vi "Actor Core.vi"(8 "error in":errorcluster, 11 "Camera Controller in":refnum<class "Camera Controller.lvclass">) -> (0 "error out":errorcluster, 3 "Actor out":refnum<class "Actor.lvclass">)   [LabVIEW 2019, in "Camera Controller.lvlib" / "Camera Controller.lvclass"]
doc: "(<B>Filename</B>: Actor Framework.lvlib:Actor.lvclass:Actor Core.vi)\n\nReceives messages to the actor, reacts to them, and initiates any error handling that may shut the actor down.\n\nDescendant classes may override this VI to append parallel tasks for the actor to complete while it handles messages. Overrides use the Call Parent Method node."
uses:
  Camera Controller.lvclass
  <vilib>/vision/Image Controls.llb/IMAQ Image.ctl
  <vilib>/ActorFramework/Message Enqueuer/Message Enqueuer.lvclass
  TypeDef/Output Data.ctl
  TypeDef/CameraControllerParameters.ctl
  TypeDef/Initialize Data CC.ctl
  <vilib>/ActorFramework/Actor/Actor.lvclass
  Image Acquisition/Image Acquisition/Image Acquisition.lvclass
  Image Acquisition/Image Acquisition Messages/Image Acqusition Setup IA Msg/Image Acqusition Setup IA Msg.lvclass
  Image Acquisition/Image Acquisition Messages/Part Name IA Msg/Part Name IA Msg.lvclass
  Image Acquisition/Image Acquisition Messages/Run IA Msg/Run IA Msg.lvclass
  Image Acquisition/Image Acquisition Messages/State Message IA Msg/State Message IA Msg.lvclass
  <vilib>/ActorFramework/Message Enqueuer/Message Priority.ctl
  <vilib>/ActorFramework/Stop Msg/Stop Msg.lvclass
  SubVI/Image Trigger Global Count.vi
  Image Acquisition/Image Acquisition Messages/Camera Setup IA Msg/Camera Setup IA Msg.lvclass
  C:/Program Files/National Instruments/LabVIEW 2019/vi.lib/ActorFramework/Actor/Actor.lvclass
panel:
  out "Camera Controller ID":i32
  out "Error Message":string
  out "Image Array Counter":u64
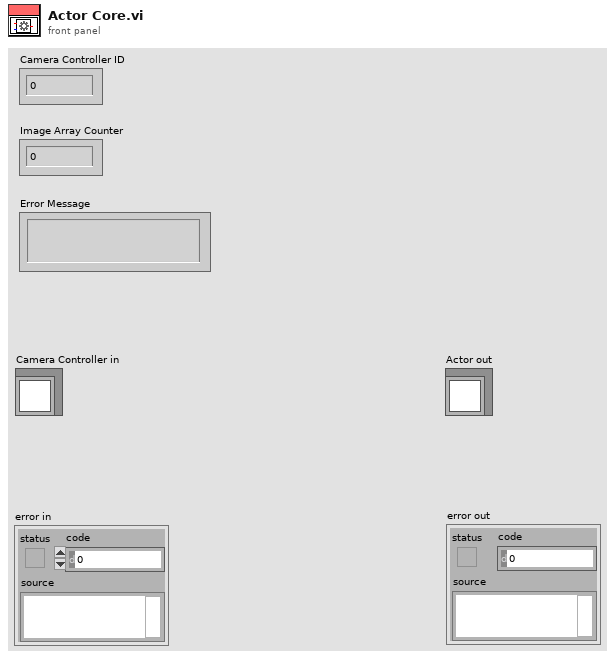
[diagram p1: front panel]
types:
  T1 = enum32{"invalid app kind", "Development System", "Run Time System", "Student Edition", "Embedded LabVIEW", "Evaluation", "Custom"}
  T2 = cluster{"Camera Id":i32, "Camera Name":string, "Exposure Time":i32, "AOI":i32[]}
  T3 = enum32{"Invalid", "Standard", "Closed", "Hidden", "Minimized", "Maximized"}
  T4 = typedef "Actor Framework.lvlib/Message Enqueuer.lvclass/Message Priority.ctl" = enum16{"Low", "Normal", "High"}
  T5 = cluster{"State":string, "Image File path":cluster{"Path":path, "Camera ID":i32}[]}
  T6 = cluster{"Image Acquisition ID":i32, "IA JSON File Path":path}
  T7 = typedef "Camera Controller.lvlib/Camera Controller.lvclass/Initialize Data CC.ctl" = cluster{"Core":cluster{"Current VI Reference":refnum<vi>, "Close Panel on Exit?":bool}, "CC ID":i32, "Part name":string, "Number of active cameras":i32[], "IA Camera names":string[], "Image count array":i32[][], "Diagnostics Child ID":i32, "Number of cameras":i32, "Image array":T8[][], "LiveMode":bool, "RecieversID":i32[], "Active Camera ID":i32[], "Enqueuer":cluster{"Caller Enqueuer":refnum<class "Message Enqueuer.lvclass">, "Nested Actor's Enqueuer":refnum<class "Message Enqueuer.lvclass">[], "Reciever Enqueuer ":cluster{"Reciever Enqueuers":refnum<class "Message Enqueuer.lvclass">, "Recievers Name":string, "Recievers ID":i32}[]}, "Image Array Counter":u64, "Images Recieved count":u64[], "All Camera Diagnostics":bool, "Output Data":T9, "Camera Setup":cluster{"Camera ID":i32, "Exposure time":i32}[], "Setup Response Received Count":u64, "Send Error to Caller":bool, "Camera Info Recieved":i32, "CameraControllerParameters":T10, "CurrentPartDetails":cluster{"PartName":string, "CameraIDs":i32[], "ReceiverSequence":cluster{"ReceiverName":string, "ReceiverID":i32, "NoOfActiveCameras":i32}[]}, "Run Info":cluster{"State":string, "Image File path":cluster{"Path":path, "Camera ID":i32}[]}, "Active Light Camera Name":string, "Captured Image Info":cluster{"Image out":T8, "Camera Location":string, "Count":u64, "RecieverSequence":cluster{"RecieverID":dbl, "Index":dbl}[]}, "Current Steps":string, "CurrentReceiverSequence":cluster{"ReceiverName":string, "ReceiverID":i32, "NoOfActiveCameras":i32}[], "Status Ack":cluster{"State":string, "Status":string}[]}
  T8 = typedef "IMAQ Image.ctl" = refnum<image>
  T9 = typedef "Camera Controller.lvlib/Camera Controller.lvclass/Output Data.ctl" = cluster{"Launch Handshake":cluster{"Actor Enqueuer Refnum":refnum<class "Message Enqueuer.lvclass">, "Actor core Refnum":refnum<vi>, "Actor Name":string}, "Launch Clear":bool, "Part Name":string, "Image Trigger Count":u64, "Image Array":T8[], "CamOpticsDiagnosticsResult":cluster{"Light Camera  Name":string, "Diagnosed Image":T8, "Dust Percentage":dbl, "Result":bool}, "State Ack":cluster{"State Message":string, "Status":string}, "Error Handler":string, "Camera Information":cluster{"Camera Id":i32, "Camera Name":string, "Exposure Time":i32, "AOI":i32[]}[], "Number of Active Camera":i32}
  T10 = typedef "Camera Controller.lvlib/Camera Controller.lvclass/CameraControllerParameters.ctl" = cluster{"CameraControllerParameters":cluster{"ID":i32, "FrontPanelOpen":bool, "NoOfCameras":i32, "CameraID":i32[], "NoOfReceivers":i32, "Diagnostics":cluster{"Path":string, "LightCameraSequence":cluster{"Name":string, "CameraID":i32, "LightID":i32}[], "Delaytime":dbl, "DecisitionParameters":cluster{"Range":i32[], "AcceptancePercentage":i32[], "Comparison":string[], "AcceptableBlackBinValue":i32}, "DiagnosticReceiverSequence":cluster{"ReceiverName":string, "ReceiverID":i32}}, "PartsList":cluster{"PartName":string, "CameraIDs":i32[], "ReceiverSequence":cluster{"ReceiverName":string, "ReceiverID":i32, "NoOfActiveCameras":i32}[]}[]}, "PartName":string[]}
  T11 = cluster{"Reciever Enqueuers":refnum<class "Message Enqueuer.lvclass">, "Recievers Name":string, "Recievers ID":i32}[]
  T12 = cluster{"Reciever Enqueuers":refnum<class "Message Enqueuer.lvclass">, "Reciever Name":string, "Reciever ID":i32}
  T13 = cluster{"Camera Id":i32, "Camera Name":string, "Exposure Time":i32, "AOI":i32[]}[]
  T14 = cluster{"ReceiverName":string, "ReceiverID":i32, "NoOfActiveCameras":i32}[]
  T15 = cluster{"ReceiverName":string, "ReceiverID":i32, "NoOfCameras":i32}
  T16 = cluster{"PartName":string, "CameraIDs":i32[], "ReceiverSequence":cluster{"ReceiverName":string, "ReceiverID":i32, "NoOfActiveCameras":i32}[]}[]
  T17 = cluster{"PartName":string, "CameraIDs":i32[], "ReceiverSequence":cluster{"ReceiverName":string, "ReceiverID":i32, "NoOfActiveCameras":i32}[]}
  T18 = cluster{"ReceiverName":string, "ReceiverID":i32, "NoOfCameras":i32}[]
  T19 = cluster{"Name":string, "CameraID":i32, "LightID":i32}[]
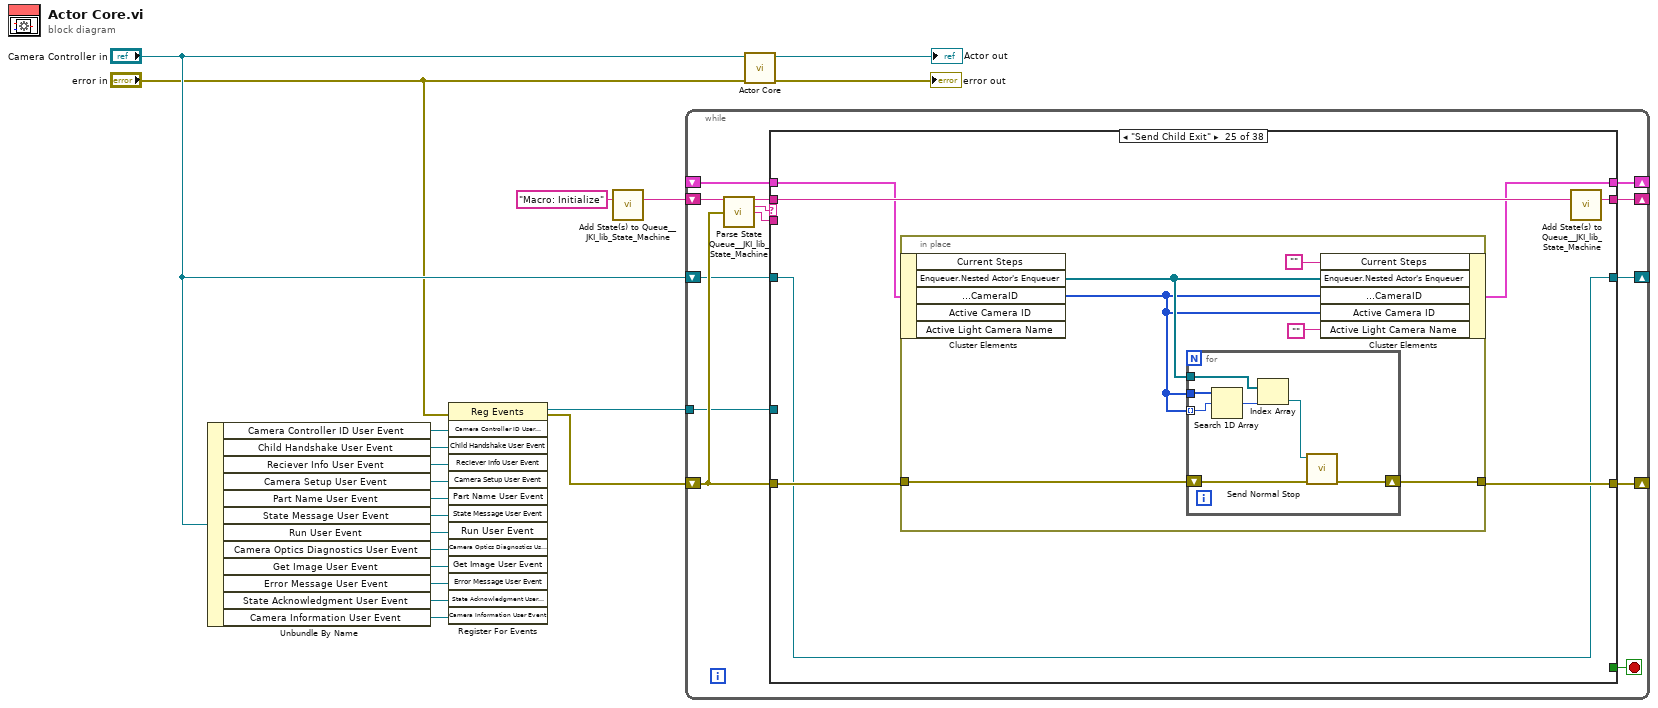
[diagram p0: block diagram]
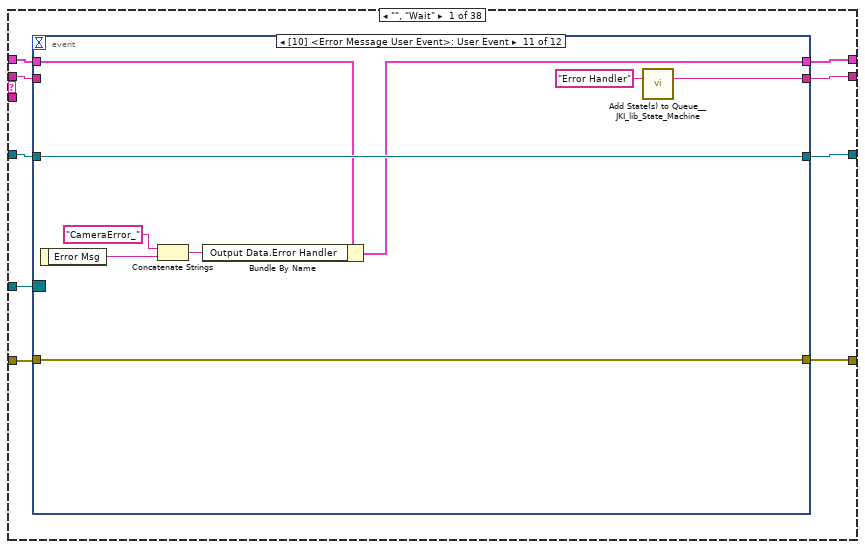
[diagram p2: hidden frame]
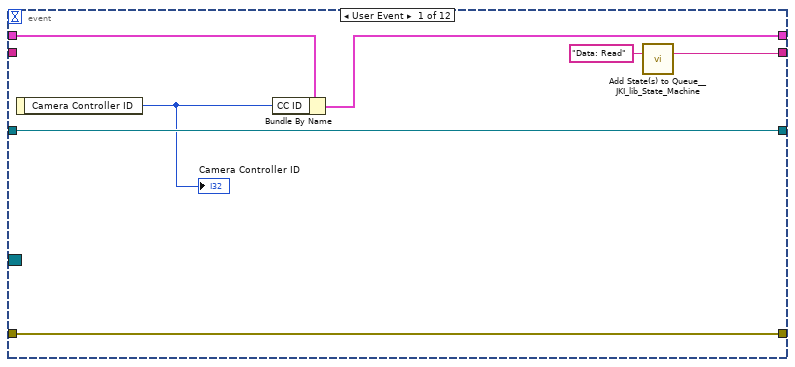
[diagram p3: hidden frame]
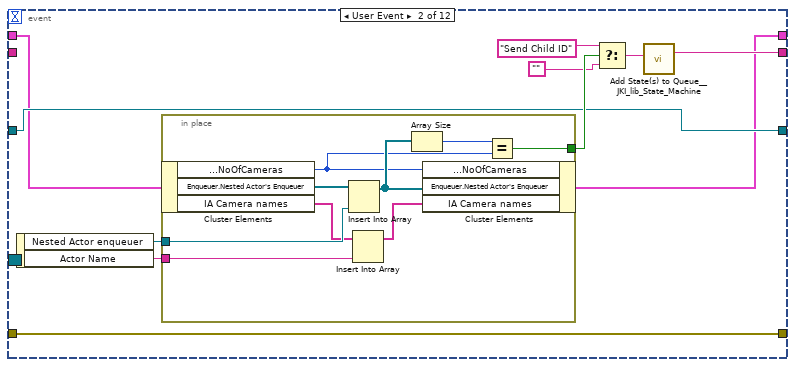
[diagram p4: hidden frame]
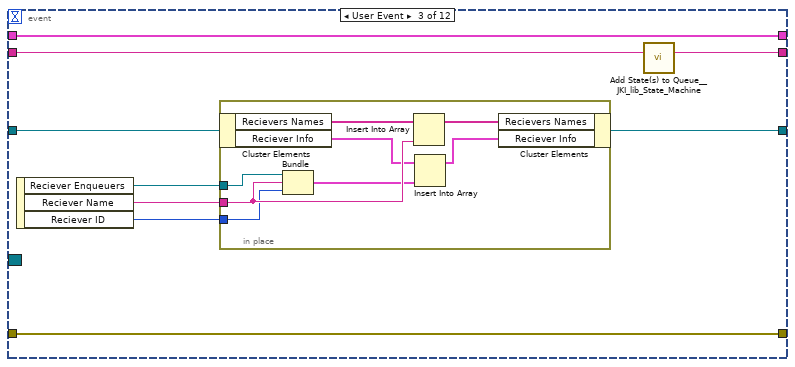
[diagram p5: hidden frame]
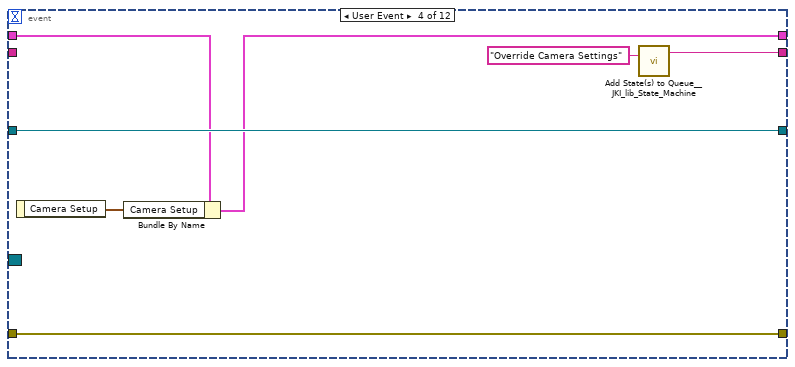
[diagram p6: hidden frame]
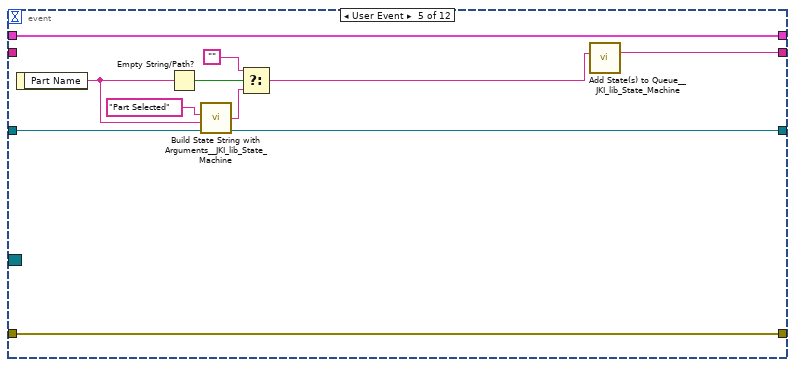
[diagram p7: hidden frame]
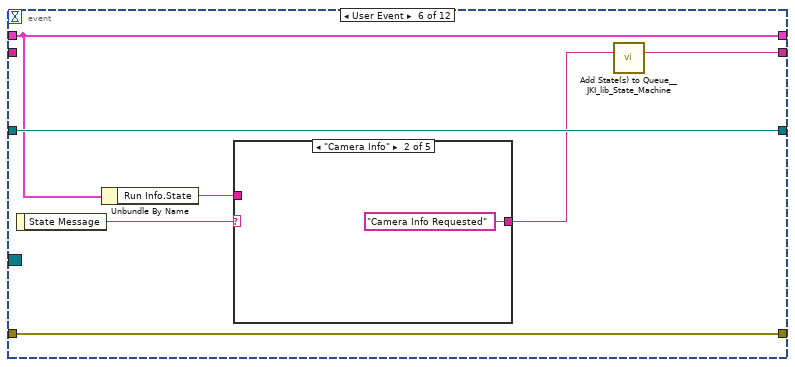
[diagram p8: hidden frame]
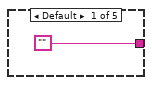
[diagram p9: hidden frame]
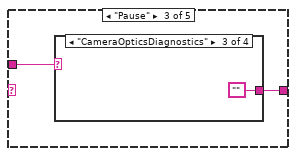
[diagram p10: hidden frame]
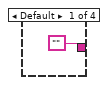
[diagram p11: hidden frame]
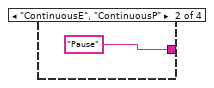
[diagram p12: hidden frame]
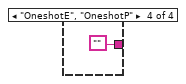
[diagram p13: hidden frame]
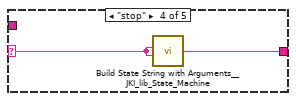
[diagram p14: hidden frame]
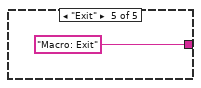
[diagram p15: hidden frame]
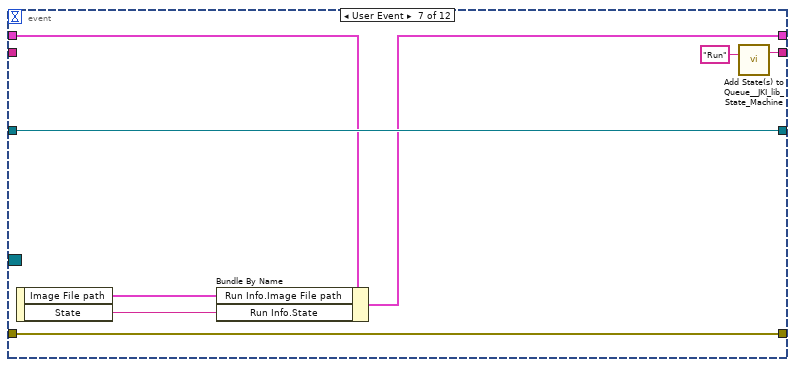
[diagram p16: hidden frame]
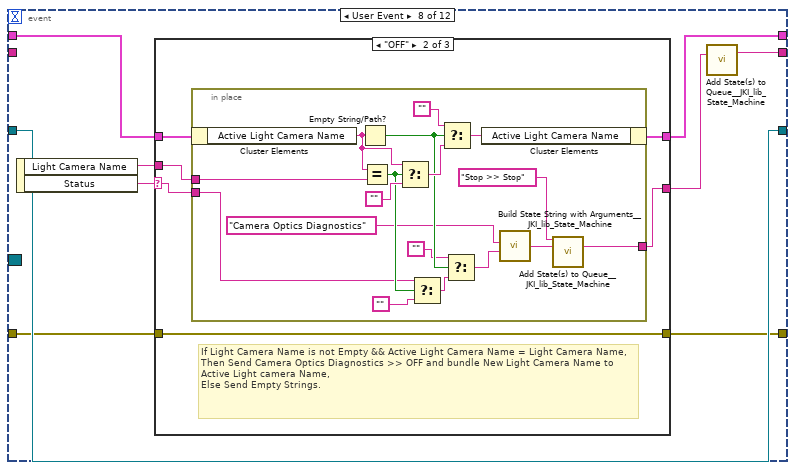
[diagram p17: hidden frame]
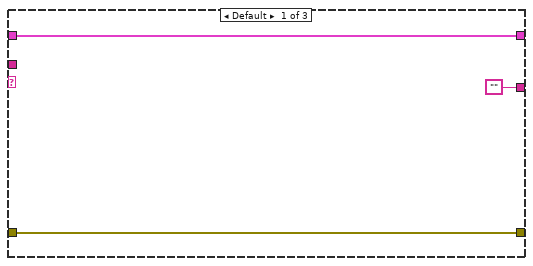
[diagram p18: hidden frame]
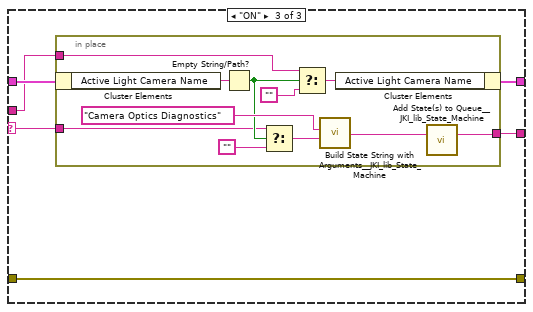
[diagram p19: hidden frame]
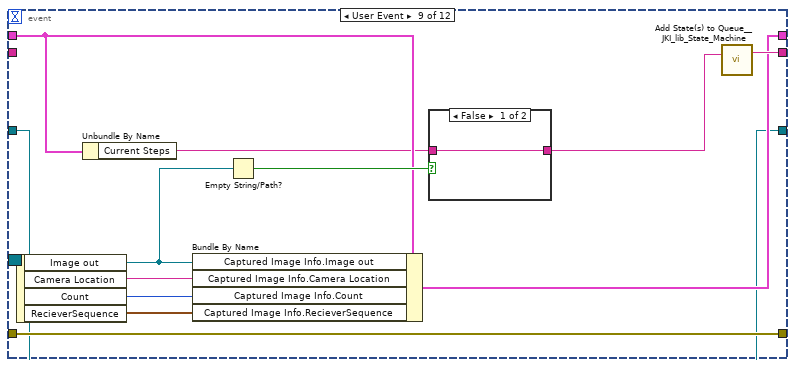
[diagram p20: hidden frame]
diagram:
  n1 = Unbundle By Name("Camera Controller in") -> ("Camera Controller ID User Event"=w16:refnum<user-event>, "Child Handshake User Event"=w15:refnum<user-event>, "Reciever Info User Event"=w14:refnum<user-event>, "Camera Setup User Event"=w13:refnum<user-event>, "Part Name User Event"=w12:refnum<user-event>, "State Message User Event"=w11:refnum<user-event>, "Run User Event"=w10:refnum<user-event>, "Camera Optics Diagnostics User Event"=w9:refnum<user-event>, "Get Image User Event"=w8:refnum<user-event>, "Error Message User Event"=w7:refnum<user-event>, "State Acknowledgment User Event"=w6:refnum<user-event>, "Camera Information User Event"=w1:refnum<user-event>)
  n2 = register-events(error in="error in", w16, w15, w14, w13, w12, w11, w10, w9, w8, w7, w6, w1) -> (reference out=w4:refnum<event-registration>, error out=w5:errorcluster)  [unwired: 1 in]
  n3 = call <vilib>:"Add State(s) to Queue__JKI_lib_State_Machine.vi"("State(s) in (\"\")"="Macro: Initialize") -> ("States Out"=w19:string)  [unwired: 14 in]
  n4 = while {
    shift-right: [w26] -> _
    shift-left: _ -> [w25]
    shift-right: [w29] -> _
    shift-left: w5 -> [w24]
    shift-right: [w28] -> _
    shift-left: w19 -> [w30]
    tunnel: w4 -> [w23]
    shift-right: [w21] -> _
    shift-left: "Camera Controller in" -> [w22]
    stop <- w27 stop-if-true
    n5 = call <vilib>:"Parse State Queue__JKI_lib_State_Machine.vi"("State Queue"=w30, "Error In (no error)"=w24) -> ("Remaining States"=w32:string, "Current State"=w33:string, "Arguments"=w31:string)  [unwired: 11 in]
    n6 = case shown="\"Send Child Exit\"" w33 {
      selector: w33 -> [_ _ w255 _ _ _ _ _ _ _ _ _ _ _ _ _ _ _ _ _ _ _ _ _ _ _ _ _ _ _ _ _ _ _ _ _ _ _]
      tunnel: w32 -> [w42 w253 w259 w278 w289 w307 w312 w317 _ w356 w361 w366 w373 w385 w412 w418 w431 w436 w443 w483 w509 _ w571 w595 w629 w647 w659 w675 _ w712 w717 _ w762 w767 _ w790 w806 w828]
      tunnel: w31 -> [_ _ _ _ _ _ _ _ _ _ _ _ w368 w379 _ _ _ _ _ w459 _ _ _ w591 _ _ _ _ _ _ _ w719 _ _ _ _ _ _]
      tunnel: w25 -> [w40 w250 w257 w269 w282 w305 w309 _ w325 w352 w358 w364 w371 w381 w409 w415 w429 w433 w439 w464 w504 w535 w566 w592 w625 w644 w648 w662 w691 w705 w714 w722 w753 w764 w773 w787 w799 w821]
      tunnel: [w39 w251 w261 w275 errorcluster {"status"=FALSE, "code"=0, "source"=""} ("error out") w304 w310 w314 w330 w351 w359 w363 w369 w382 w410 w416 w420 w434 w440 w465 w506 w536 w568 w593 w626 w645 w656 w672 w692 w709 w715 w720 w750 w765 w776 w788 w803 w825] -> w29
      tunnel: w24 -> [w38 w251 w260 w275 w281 w304 w310 w314 w331 w353 w359 w363 w370 w383 w410 w416 w421 w434 w441 w466 w507 w537 w569 w589 w627 w645 w657 w673 w693 w710 w715 w720 w754 w765 w777 w788 w804 w826]
      tunnel: [w41 w252 w258 w277 w288 w306 w311 w316 w332 w355 w360 w365 w372 w384 w411 w417 w430 w435 w442 w482 w508 w538 w570 w594 w628 w646 w658 w674 w694 w711 w716 w724 w761 w766 w778 w789 w805 w827] -> w28
      tunnel: [_ _ _ _ _ TRUE _ _ _ _ _ _ _ _ _ _ _ _ _ _ _ _ _ _ _ _ _ _ _ _ _ _ _ _ _ _ _ _] -> w27
      tunnel: [w37 w250 w257 w276 w282 w305 w309 w315 w324 w352 w358 w364 w371 w381 w409 w415 w429 w433 w438 w477 w503 w534 w565 w586 w624 w644 w648 w661 w691 w705 w714 w721 w753 w764 w772 w787 w798 w820] -> w26
      tunnel: w23 -> [w36 _ _ _ _ _ _ _ _ w346 _ _ _ _ _ _ w419 _ _ _ _ _ _ w587 _ _ _ _ _ _ _ _ _ _ _ _ _ _]
      tunnel: w22 -> [w35 w249 w254 w266 w285 w302 w308 w313 w329 w350 w357 w362 w367 w378 w408 w413 w422 w432 w437 w478 w505 w533 w567 w590 w623 w643 w650 w660 w688 w708 w713 w723 w749 w763 w774 w786 w802 w824]
      tunnel: [w34 w249 w254 w266 w284 w302 w308 w313 w329 w349 w357 w362 w367 w378 w408 w413 w422 w432 w437 w478 w505 w533 w567 w590 w623 w643 w649 w660 w688 w707 w713 w723 w748 w763 w775 w786 w801 w823] -> w21
      frame "", "Wait" {
        n7 = event shown="[10] <Error Message User Event>: User Event" {
          selector: w36 -> [_ _ _ _ _ _ _ _ _ _ _ _]
          dyn-events: _ -> [_ _ _ _ _ _ _ _ _ _ _ _]
          timeout: _ -> [_ _ _ _ _ _ _ _ _ _ _ _]
          tunnel: w42 -> [_ _ w75 _ _ _ _ _ _ _ _ w235]
          tunnel: [w49 w59 w76 w92 w101 w109 w129 w138 w192 w197 w226 w236] -> w41
          tunnel: w40 -> [w44 w51 w77 w89 w102 w105 w126 w134 w184 w199 w223 w234]
          tunnel: [w48 w60 w78 w93 w103 w110 w127 w130 w193 w206 w227 w237] -> w39
          tunnel: w38 -> [w48 w60 w78 w93 w103 w110 w127 w131 w193 w206 w227 w237]
          tunnel: [w43 w50 w77 w88 w102 w105 w123 w133 w188 w198 w222 w233] -> w37
          tunnel: w35 -> [w46 w52 w74 w91 w100 w108 w128 w132 w186 w205 w225 w228]
          tunnel: [w46 w52 w70 w91 w100 w108 w128 w132 w186 w205 w225 w228] -> w34
          event User Event {
            n8 = event-data() -> ("Camera Controller ID"=w45:i32)  [unwired: 1 in]
            "Camera Controller ID" <- w45
            n9 = Bundle By Name(cluster=w44, "CC ID"=w45) -> (w43:T7)
            n10 = call <vilib>:"Add State(s) to Queue__JKI_lib_State_Machine.vi"("State(s) in (\"\")"="Data: Read" ("State(s) in (\"\")")) -> ("States Out"=w49:string)  [unwired: 14 in]
          }
          event User Event {
            n11 = event-data() -> ("Nested Actor enqueuer"=w58:refnum<class "Message Enqueuer.lvclass">, "Actor Name"=w57:string)  [unwired: 1 in]
            n12 = in-place {
              in-place-border: w58 -> [w68]
              in-place-border: w57 -> [w66]
              in-place-border: [w61] -> w56
              n13 = in-place-cluster #1(w51) -> ("CameraControllerParameters.CameraControllerParameters.NoOfCameras"=w62:i32, "Enqueuer.Nested Actor's Enqueuer"=w69:refnum<class "Message Enqueuer.lvclass">[], "IA Camera names"=w67:string[])
              n14 = Insert Into Array(array=w69, new element=w68) -> (w63:refnum<class "Message Enqueuer.lvclass">[])  [unwired: 1 in]
              n15 = Insert Into Array(array=w67, new element=w66) -> (w65:string[])  [unwired: 1 in]
              n16 = Array Size(array=w63) -> (size(s)=w64:i32)
              n17 = in-place-cluster #1("CameraControllerParameters.CameraControllerParameters.NoOfCameras"=w62, "Enqueuer.Nested Actor's Enqueuer"=w63, "IA Camera names"=w65) -> (w50:T7)
              n18 = Equal?(x=w64, y=w62) -> (x = y?=w61:bool)
            }
            n19 = Select(t="Send Child ID", s=w56, f="") -> (s? t:f=w55:string)
            n20 = call <vilib>:"Add State(s) to Queue__JKI_lib_State_Machine.vi"("State(s) in (\"\")"=w55) -> ("States Out"=w59:string)  [unwired: 14 in]
          }
          event User Event {
            n21 = event-data() -> ("Reciever Enqueuers"=w73:refnum<class "Message Enqueuer.lvclass">, "Reciever Name"=w72:string, "Reciever ID"=w71:i32)  [unwired: 1 in]
            n22 = in-place {
              in-place-border: w73 -> [w84]
              in-place-border: w72 -> [w83]
              in-place-border: w71 -> [w82]
              n23 = in-place-cluster #2(w74) -> ("Recievers Names"=w86:string[], "Reciever Info"=w80:T11)
              n24 = Bundle("Reciever Enqueuers"=w84, "Reciever Name"=w83, "Reciever ID"=w82) -> (w81:T12)  [unwired: 1 in]
              n25 = Insert Into Array(array=w86, new element=w83) -> (w85:string[])  [unwired: 1 in]
              n26 = Insert Into Array(array=w80, new element=w81) -> (w79:T11)  [unwired: 1 in]
              n27 = in-place-cluster #2("Recievers Names"=w85, "Reciever Info"=w79) -> (w70:refnum<class "Camera Controller.lvclass">)
            }
            n28 = call <vilib>:"Add State(s) to Queue__JKI_lib_State_Machine.vi"("State(s) in (\"\")"=w75) -> ("States Out"=w76:string)  [unwired: 14 in]
          }
          event User Event {
            n29 = event-data() -> ("Camera Setup"=w90:cluster{"Camera ID":i32, "Exposure time":i32}[])  [unwired: 1 in]
            n30 = Bundle By Name(cluster=w89, "Camera Setup"=w90) -> (w88:T7)
            n31 = call <vilib>:"Add State(s) to Queue__JKI_lib_State_Machine.vi"("State(s) in (\"\")"="Override Camera Settings" ("State(s) in (\"\")")) -> ("States Out"=w92:string)  [unwired: 14 in]
          }
          event User Event {
            n32 = event-data() -> ("Part Name"=w96:string)  [unwired: 1 in]
            n33 = Empty String/Path?(string/path=w96) -> (empty?=w98:bool)
            n34 = call <vilib>:"Build State String with Arguments__JKI_lib_State_Machine.vi"("Arguments (\"\")"=w96, "State"="Part Selected" ("State(s) in (\"\")")) -> ("State with Arguments"=w97:string)  [unwired: 4 in]
            n35 = Select(t="", s=w98, f=w97) -> (s? t:f=w94:string)
            n36 = call <vilib>:"Add State(s) to Queue__JKI_lib_State_Machine.vi"("State(s) in (\"\")"=w94) -> ("States Out"=w101:string)  [unwired: 14 in]
          }
          event User Event {
            n37 = event-data() -> ("State Message"=w107:string)  [unwired: 1 in]
            n38 = Unbundle By Name(w105) -> ("Run Info.State"=w104:string)
            n39 = case shown="\"Camera Info\"" w107 {
              selector: w107 -> [_ _ _ w119 _]
              tunnel: ["" "Camera Info Requested" ("State with Arguments") w113 w120 "Macro: Exit"] -> w106
              tunnel: w104 -> [_ _ w114 _ _]
              frame Default {
              }
              frame "Camera Info" {
              }
              frame "Pause" {
                n40 = case shown="\"CameraOpticsDiagnostics\"" w114 {
                  tunnel: ["" "Pause" "" ""] -> w113
                  frame Default {
                  }
                  frame "ContinuousE", "ContinuousP" {
                  }
                  frame "CameraOpticsDiagnostics" {
                  }
                  frame "OneshotE", "OneshotP" {
                  }
                }
              }
              frame "stop" {
                n41 = call <vilib>:"Build State String with Arguments__JKI_lib_State_Machine.vi"("Arguments (\"\")"=w119, "State"=w119) -> ("State with Arguments"=w120:string)  [unwired: 4 in]
              }
              frame "Exit" {
              }
            }
            n42 = call <vilib>:"Add State(s) to Queue__JKI_lib_State_Machine.vi"("State(s) in (\"\")"=w106) -> ("States Out"=w109:string)  [unwired: 14 in]
          }
          event User Event {
            n43 = event-data() -> ("Image File path"=w124:cluster{"Path":path, "Camera ID":i32}[], "State"=w125:string)  [unwired: 1 in]
            n44 = Bundle By Name(cluster=w126, "Run Info.Image File path"=w124, "Run Info.State"=w125) -> (w123:T7)
            n45 = call <vilib>:"Add State(s) to Queue__JKI_lib_State_Machine.vi"("State(s) in (\"\")"="Run" ("State(s) in (\"\")")) -> ("States Out"=w129:string)  [unwired: 14 in]
          }
          event User Event {
            n46 = event-data() -> ("Light Camera Name"=w136:string, "Status"=w135:string)  [unwired: 1 in]
            n47 = case shown="\"OFF\"" w135 {
              selector: w135 -> [_ w143 w167]
              tunnel: ["" w144 w166] -> w137
              tunnel: w134 -> [w141 w147 w170]
              tunnel: w136 -> [_ w146 w169]
              tunnel: [w141 w145 w168] -> w133
              tunnel: w131 -> [w139 w142 w165]
              tunnel: [w139 w142 w165] -> w130
              frame Default {
              }
              frame "OFF" {
                # "If Light Camera Name is not Empty && Active Light Camera Name = Light Camera Name,\nThen Send Camera Optics Diagnostics >> OFF and bundle New Light Camera Name to Active Light camera Name, \nElse Send Empty Strings."
                n48 = in-place {
                  in-place-border: w146 -> [w163]
                  in-place-border: [w148] -> w144
                  in-place-border: w143 -> [w153]
                  n49 = in-place-cluster #3(w147) -> ("Active Light Camera Name"=w160:string)
                  n50 = Empty String/Path?(string/path=w160) -> (empty?=w158:bool)
                  n51 = Equal?(x=w160, y=w163) -> (x = y?=w157:bool)
                  n52 = Select(t=w160, s=w157, f="") -> (s? t:f=w161:string)
                  n53 = Select(t=w153, s=w157, f="") -> (s? t:f=w156:string)
                  n54 = Select(t="" ("f"), s=w158, f=w161) -> (s? t:f=w162:string)
                  n55 = Select(t="" ("f"), s=w158, f=w156) -> (s? t:f=w152:string)
                  n56 = in-place-cluster #3("Active Light Camera Name"=w162) -> (w145:T7)
                  n57 = call <vilib>:"Build State String with Arguments__JKI_lib_State_Machine.vi"("Arguments (\"\")"=w152, "State"="Camera Optics Diagnostics" ("State(s) in (\"\")")) -> ("State with Arguments"=w150:string)  [unwired: 4 in]
                  n58 = call <vilib>:"Add State(s) to Queue__JKI_lib_State_Machine.vi"("State(s) in Front (\"\")"="Stop >> Stop" ("State(s) in (\"\")"), "State(s) in (\"\")"=w150) -> ("States Out"=w148:string)  [unwired: 13 in]
                }
              }
              frame "ON" {
                n59 = in-place {
                  in-place-border: w169 -> [w180]
                  in-place-border: w167 -> [w175]
                  in-place-border: [w171] -> w166
                  n60 = in-place-cluster #4(w170) -> ("Active Light Camera Name"=w181:string)
                  n61 = Empty String/Path?(string/path=w181) -> (empty?=w176:bool)
                  n62 = Select(t=w175, s=w176, f="") -> (s? t:f=w173:string)
                  n63 = Select(t=w180, s=w176, f="") -> (s? t:f=w178:string)
                  n64 = call <vilib>:"Build State String with Arguments__JKI_lib_State_Machine.vi"("Arguments (\"\")"=w173, "State"="Camera Optics Diagnostics" ("State(s) in (\"\")")) -> ("State with Arguments"=w172:string)  [unwired: 4 in]
                  n65 = in-place-cluster #4("Active Light Camera Name"=w178) -> (w168:T7)
                  n66 = call <vilib>:"Add State(s) to Queue__JKI_lib_State_Machine.vi"("State(s) in (\"\")"=w172) -> ("States Out"=w171:string)  [unwired: 14 in]
                }
              }
            }
            n67 = call <vilib>:"Add State(s) to Queue__JKI_lib_State_Machine.vi"("State(s) in (\"\")"=w137) -> ("States Out"=w138:string)  [unwired: 14 in]
          }
          event User Event {
            n68 = event-data() -> ("Image out"=w187:T8, "Camera Location"=w191:string, "Count"=w190:u64, "RecieverSequence"=w189:cluster{"RecieverID":dbl, "Index":dbl}[])  [unwired: 1 in]
            n69 = Unbundle By Name(w184) -> ("Current Steps"=w183:string)
            n70 = Bundle By Name(cluster=w184, "Captured Image Info.Image out"=w187, "Captured Image Info.Camera Location"=w191, "Captured Image Info.Count"=w190, "Captured Image Info.RecieverSequence"=w189) -> (w188:T7)
            n71 = Empty String/Path?(string/path=w187) -> (empty?=w185:bool)
            n72 = case shown="False" w185 {
              tunnel: w183 -> [w194 _]
              tunnel: [w194 ""] -> w182
              frame False {
              }
              frame True {
              }
            }
            n73 = call <vilib>:"Add State(s) to Queue__JKI_lib_State_Machine.vi"("State(s) in (\"\")"=w182) -> ("States Out"=w192:string)  [unwired: 14 in]
          }
          event User Event {
            n74 = event-data() -> ("Camera Id"=w201:i32, "Camera Name"=w204:string, "Exposure Time"=w202:i32, "AOI"=w203:i32[])  [unwired: 1 in]
            n75 = Bundle("Camera Id"=w201, "Camera Name"=w204, "Exposure Time"=w202, "AOI"=w203) -> (w200:T2)  [unwired: 1 in]
            n76 = in-place {
              in-place-border: w201 -> [w216]
              in-place-border: w200 -> [w217]
              in-place-border: [w208] -> w196
              n77 = in-place-cluster #5(w199) -> ("Active Camera ID"=w213:i32[], "Camera Info Recieved"=w212:i32, "Output Data.Camera Information"=w218:T13)
              n78 = Array Size(array=w213) -> (size(s)=w214:i32)
              n79 = Increment(x=w212) -> (x+1=w211:i32)
              n80 = Replace Array Subset(array=w218, new element=w217, index=w216) -> (w215:T13)
              n81 = Equal?(x=w214, y=w211) -> (x = y?=w210:bool)
              n82 = Select(t="Send Merged Camera Information", s=w210, f="") -> (s? t:f=w208:string)
              n83 = in-place-cluster #5("Active Camera ID"=w213, "Camera Info Recieved"=w211, "Output Data.Camera Information"=w215) -> (w198:T7)
            }
            n84 = call <vilib>:"Add State(s) to Queue__JKI_lib_State_Machine.vi"("State(s) in (\"\")"=w196) -> ("States Out"=w197:string)  [unwired: 14 in]
          }
          event User Event {
            n85 = event-data() -> ("Error Msg"=w220:string)  [unwired: 1 in]
            n86 = Concatenate Strings("CameraError_" ("string"), w220) -> (w219:string)
            n87 = Bundle By Name(cluster=w223, "Output Data.Error Handler"=w219) -> (w222:T7)
            n88 = call <vilib>:"Add State(s) to Queue__JKI_lib_State_Machine.vi"("State(s) in (\"\")"="Error Handler" ("State(s) in (\"\")")) -> ("States Out"=w226:string)  [unwired: 14 in]
          }
          event User Event {
            n89 = event-data() -> ("State"=w231:string, "Status"=w232:string)  [unwired: 1 in]
            n90 = Bundle("State"=w231, "Status"=w232) -> (w230:cluster{"State":string, "Status":string})  [unwired: 1 in]
            n91 = in-place {
              in-place-border: w230 -> [w238]
              in-place-border: [w240] -> w229
              n92 = in-place-cluster #6(w234) -> ("Active Camera ID"=w245:i32[], "Setup Response Received Count"=w244:u64, "Status Ack"=w248:cluster{"State":string, "Status":string}[])
              n93 = Array Size(array=w245) -> (size(s)=w246:i32)
              n94 = Increment(x=w244) -> (x+1=w243:u64)
              n95 = Replace Array Subset(array=w248, new element=w238) -> (w247:cluster{"State":string, "Status":string}[])  [unwired: 1 in]
              n96 = Equal?(x=w246, y=w243) -> (x = y?=w242:bool)
              n97 = Select(t="Send State Ack", s=w242, f="") -> (s? t:f=w240:string)
              n98 = in-place-cluster #6("Active Camera ID"=w245, "Setup Response Received Count"=w243, "Status Ack"=w247) -> (w233:T7)
            }
            n99 = call <vilib>:"Add State(s) to Queue__JKI_lib_State_Machine.vi"("State(s) in Front (\"\")"=w229, "State(s) in (\"\")"=w235) -> ("States Out"=w236:string)  [unwired: 13 in]
          }
        }
      }
      frame "---------- Core ----------" {
        n100 = call <vilib>:"Add State(s) to Queue__JKI_lib_State_Machine.vi"("State(s) in (\"\")"=w253) -> ("States Out"=w252:string)  [unwired: 14 in]
      }
      frame Default {
        w264 = 42 items=["No error", "Argument error", "Memory is full", "Out of zone", "End of file", "File already open", "Generic file I/O error", "File not found", "File permission error", "Disk is full", "Duplicate path", "Too many files open", "System feature not enabled", "Resource file not found", "Cannot add resource", "Resource not found", "Image not found", "Image memory error", "Pen does not exist", "Config type invalid", "Config token not found", "Config parse error", "Config memory error", "Bad external code format", "Bad external code offset", "External code not present", "Null window", "Destroy window error", "Null menu", "Print aborted", "Bad print record", "Print driver error", "Windows error during printing", "Memory error during printing", "Print dialog error", "Generic print error", "Invalid device refnum", "Device not found", "Device parameter error", "Device unit error", "Cannot open device", "Device call aborted", "Generic error", "Cancelled by user", "Object ID too low", "Object ID too high", "Object not in heap", "Unknown heap", "Unknown object (invalid DefProc)", "Unknown object (DefProc not in table)", "Message out of range", "Invalid (null) method", "Unknown message", "Manager call not supported", "Bad address", "Network operation in progress", "Network operation timed out", "Connection is busy", "Network attribute not supported", "Network error", "Address in use", "System out of memory", "Connection aborted", "Connection refused", "Not connected", "Already connected", "Connection closed", "Initialization error (interapplication manager)", "Bad occurrence", "Wait on unbound occurrence handler", "Occurrence queue overflow", "Datalog type conflict", "Unused", "Unrecognized type (interapplication manager)", "Memory corrupt", "Failed to make temporary DLL", "Old CIN version", "Drag socket not found", "Failed to load drop-object", "Failed to register OLE object", "Failed to release OLE object", "Format specifier type mismatch", "Unknown format specifier", "Too few format specifiers", "Too many format specifiers", "Scan failed", "Newer CIN version", "Error converting to variant", "Runtime menu error", "Password tampered", "Variant attribute not found", "Incompatible variant data type", "Event data is not available", "Event Store is not present", "Occurrence is not found", "Event Queue is not created", "Event info is not available", "Refnum passed is NULL", "Error retrieving Class GUID", "Error retrieving CoClass GUID", "Error retrieving TypeLib GUID.", "Bad built application magic bytes.", "Specific driver is different from the specific driver associated with the Logical Name.", "There is no session opened to the class driver.", "Max Error", "MAX - Error with config objects", "MAX - Error loading configuration", "MAX - Group not supported"]
        # "Current State"
        # "Do not delete, rename, or modify this frame.\n(this is used to capture unhandled states and typos)"
        # "Handle mistyped state name (developer tool)"
        n101 = Format Into String(format string="Software Exception: Unhandled State \"%s\"." ("message"), error in=w260, w255) -> (resulting string=w263:string, error out=w262:errorcluster)  [unwired: 1 in]
        n102 = call <vilib>:"Error Cluster From Error Code.vi"("show call chain? (False)"=TRUE, "error in (no error)"=w262, "error message (\"\")"=w263, "error code (0)"=w264) -> ("error out"=w261:errorcluster)  [unwired: 5 in]
        n103 = call <vilib>:"Add State(s) to Queue__JKI_lib_State_Machine.vi"("State(s) in (\"\")"=w259) -> ("States Out"=w258:string)  [unwired: 14 in]
      }
      frame "Initialize Core Data" {
        # "Do not delete, rename, or modify this frame.\n(this is used to determine panel behavior on exit)"
        # "originally closed?"
        # "exe?"
        # "If panel starts closed or is an EXE, then close it when we exit"
        n104 = property class="VI"() -> ("Front Panel.Open"=w274:bool)  [unwired: 2 in, 2 out]
        n105 = property class="App"() -> ("App.Kind"=w273:T1)  [unwired: 2 in, 2 out]
        n106 = control-ref of="Current VI Reference"() -> (w267:refnum<vi>)
        n107 = Not(x=w274) -> (.not. x?=w271:bool)
        n108 = Equal?(x=w273, y=T1."Run Time System" ("Application:Kind")) -> (x = y?=w270:bool)
        n109 = Or(x=w271, y=w270) -> (x .or. y?=w268:bool)
        n110 = Bundle By Name(cluster=w269, "Core.Current VI Reference"=w267, "Core.Close Panel on Exit?"=w268) -> (w276:T7)
        n111 = call <vilib>:"Add State(s) to Queue__JKI_lib_State_Machine.vi"("State(s) in (\"\")"=w278) -> ("States Out"=w277:string)  [unwired: 14 in]
      }
      frame "Error Handler" {
        # "Clear error"
        n112 = case shown="No Error" w281 {
          selector: w281 -> [_ w301]
          tunnel: w282 -> [w291 w299]
          tunnel: [w290 w297] -> w280
          frame No Error {
            n113 = Unbundle By Name(w291) -> ("Output Data"=w290:T9)
          }
          frame Error {
            n114 = Unbundle By Name(w301) -> ("code"=w300:i32)
            n115 = Unbundle By Name(w299) -> ("Output Data"=w298:T9)
            n116 = Number To Decimal String(number=w300) -> (decimal integer string=w294:string)  [unwired: 1 in]
            n117 = Concatenate Strings("CameraError" ("string"), "_" ("string"), "FFAX", w294) -> (w296:string)
            n118 = Bundle By Name(cluster=w298, "Error Handler"=w296) -> (w297:T9)
          }
        }
        n119 = Unbundle By Name(w280) -> ("Error Handler"=→"Error Message":string)
        n120 = call "ZenCAM Output.vi"("Output Data"=w280, "State"="Error Alert", "Camera Controller in"=w285) -> ("Camera Controller out"=w284:refnum<class "Camera Controller.lvclass">)  [unwired: 7 in, 1 out]
        n121 = call <vilib>:"Add State(s) to Queue__JKI_lib_State_Machine.vi"("State(s) in Front (\"\")"="/* Post Error States", "State(s) in (\"\")"=w289) -> ("States Out"=w288:string)  [unwired: 13 in]
      }
      frame "Exit" {
        # "Do not put any code in this frame.\n(No errors that occur here will be handled.)"
        n122 = call <vilib>:"Add State(s) to Queue__JKI_lib_State_Machine.vi"("State(s) in (\"\")"=w307) -> ("States Out"=w306:string)  [unwired: 14 in]
      }
      frame "---------- Data ----------" {
        n123 = call <vilib>:"Add State(s) to Queue__JKI_lib_State_Machine.vi"("State(s) in (\"\")"=w312) -> ("States Out"=w311:string)  [unwired: 14 in]
      }
      frame "Data: Initialize" {
        w315 = T7 {"Core"={"Current VI Reference"=refnum, "Close Panel on Exit?"=FALSE}, "CC ID"=0, "Part name"="", "Number of active cameras"=[], "IA Camera names"=[], "Image count array"=[], "Diagnostics Child ID"=-1, "Number of cameras"=0, "Image array"=[], "LiveMode"=TRUE, "RecieversID"=[], "Active Camera ID"=[], "Enqueuer"={"Caller Enqueuer"=refnum, "Nested Actor's Enqueuer"=[], "Reciever Enqueuer "=[]}, "Image Array Counter"=0, "Images Recieved count"=[], "All Camera Diagnostics"=FALSE, "Output Data"={"Launch Handshake"={"Actor Enqueuer Refnum"=refnum, "Actor core Refnum"=refnum, "Actor Name"=""}, "Launch Clear"=TRUE, "Part Name"="", "Image Trigger Count"=0, "Image Array"=[], "CamOpticsDiagnosticsResult"={"Light Camera  Name"="", "Diagnosed Image"=refnum, "Dust Percentage"=0.0, "Result"=FALSE}, "State Ack"={"State Message"="", "Status"=""}, "Error Handler"="", "Camera Information"=[], "Number of Active Camera"=0}, "Camera Setup"=[], "Setup Response Received Count"=0, "Send Error to Caller"=FALSE, "Camera Info Recieved"=0, "CameraControllerParameters"={"CameraControllerParameters"={"ID"=0, "FrontPanelOpen"=FALSE, "NoOfCameras"=0, "CameraID"=[], "NoOfReceivers"=0, "Diagnostics"={"Path"="", "LightCameraSequence"=[], "Delaytime"=0.0, "DecisitionParameters"={"Range"=[], "AcceptancePercentage"=[], "Comparison"=[], "AcceptableBlackBinValue"=0}, "DiagnosticReceiverSequence"={"ReceiverName"="", "ReceiverID"=0}}, "PartsList"=[]}, "PartName"=[]}, "CurrentPartDetails"={"PartName"="", "CameraIDs"=[], "ReceiverSequence"=[]}, "Run Info"={"State"="", "Image File path"=[]}, "Active Light Camera Name"="", "Captured Image Info"={"Image out"=refnum, "Camera Location"="", "Count"=0, "RecieverSequence"=[{"RecieverID"=0.0, "Index"=1.0}, {"RecieverID"=1.0, "Index"=2.0}]}, "Current Steps"="", "CurrentReceiverSequence"=[], "Status Ack"=[]}  # Camera Control Cluster
        n124 = call <vilib>:"Add State(s) to Queue__JKI_lib_State_Machine.vi"("State(s) in (\"\")"=w317) -> ("States Out"=w316:string)  [unwired: 14 in]
      }
      frame "Data: Read" {
        n125 = Unbundle By Name(w329) -> ("CC Json File Path"=w328:path)
        n126 = Unbundle By Name(w325) -> ("CC ID"=w327:i32)
        n127 = Number To Decimal String(number=w327) -> (decimal integer string=w326:string)  [unwired: 1 in]
        n128 = call "JSONRead.vi"("error in"=w331, "CameraController ID"=w326, "file path (use dialog)"=w328) -> ("error out"=w330:errorcluster, "Camera Controller Parameters"=w318:T10)  [unwired: 7 in]
        n129 = in-place {
          in-place-border: w318 -> [w345]
          n130 = in-place-cluster #7(w325) -> ("CurrentReceiverSequence"=w337:T14)  [unwired: 3 out]
          n131 = in-place-cluster #8(w318) -> ("CameraControllerParameters.CameraID"=w338:i32[], "CameraControllerParameters.Diagnostics.DiagnosticReceiverSequence.ReceiverName"=w342:string, "CameraControllerParameters.Diagnostics.DiagnosticReceiverSequence.ReceiverID"=w341:i32, "CameraControllerParameters.NoOfCameras"=w340:i32)
          n132 = Bundle("ReceiverName"=w342, "ReceiverID"=w341, "NoOfCameras"=w340) -> (w344:T15)  [unwired: 1 in]
          n133 = Array Size(array=w338) -> (size(s)=w334:i32)
          n134 = Insert Into Array(array=w337, new element=w344) -> (w343:T14)  [unwired: 1 in]
          n135 = Initialize Array(T2 {"Camera Id"=0, "Camera Name"="", "Exposure Time"=0, "AOI"=[]} ("Camera Information"), w334) -> (w336:T13)
          n136 = Initialize Array(cluster{"State":string, "Status":string} {"State"="", "Status"=""} ("Status Ack"), w334) -> (w333:cluster{"State":string, "Status":string}[])
          n137 = in-place-cluster #7("CameraControllerParameters"=w345, "CurrentReceiverSequence"=w343, "Output Data.Camera Information"=w336, "Status Ack"=w333) -> (w324:T7)
          n138 = in-place-cluster #8("CameraControllerParameters.CameraID"=w338, "CameraControllerParameters.Diagnostics.DiagnosticReceiverSequence.ReceiverName"=w342, "CameraControllerParameters.Diagnostics.DiagnosticReceiverSequence.ReceiverID"=w341, "CameraControllerParameters.NoOfCameras"=w340) -> ()  [unwired: 1 out]
        }
        n139 = Unbundle By Name(w318) -> ("CameraControllerParameters.FrontPanelOpen"=w323:bool)
        n140 = Select(t="UI: Front Panel State >> Open" ("State(s) in (\"\")"), s=w323, f="UI: Front Panel State >> Close" ("State(s) in (\"\")")) -> (s? t:f=w320:string)
        n141 = call <vilib>:"Add State(s) to Queue__JKI_lib_State_Machine.vi"("State(s) in Front (\"\")"=w320, "State(s) in (\"\")"="Launch Child Actor" ("State(s) in (\"\")")) -> ("States Out"=w332:string)  [unwired: 13 in]
      }
      frame "Data: Cleanup" {
        n142 = Unbundle By Name(w352) -> ("Core.Current VI Reference"=w354:refnum<vi>)
        n143 = Close Reference(reference=w354, error in (no error)=w353) -> (error out=w348:errorcluster)
        n144 = Unregister For Events(event registration refnum=w346, error in=w348) -> (error out=w347:errorcluster)
        n145 = call "Destroy User Event.vi"("error in (no error)"=w347, "Camera Controller in"=w350) -> ("error out"=w351:errorcluster, "Camera Controller out"=w349:refnum<class "Camera Controller.lvclass">)  [unwired: 8 in]
        n146 = call <vilib>:"Add State(s) to Queue__JKI_lib_State_Machine.vi"("State(s) in (\"\")"=w356) -> ("States Out"=w355:string)  [unwired: 14 in]
      }
      frame "---------- UI ----------" {
        n147 = call <vilib>:"Add State(s) to Queue__JKI_lib_State_Machine.vi"("State(s) in (\"\")"=w361) -> ("States Out"=w360:string)  [unwired: 14 in]
      }
      frame "UI: Initialize" {
        n148 = call <vilib>:"Add State(s) to Queue__JKI_lib_State_Machine.vi"("State(s) in (\"\")"=w366) -> ("States Out"=w365:string)  [unwired: 14 in]
      }
      frame "UI: Cursor Set" {
        # "Argument"
        n149 = case shown="\"Idle\", Default" w368 {
          tunnel: w370 -> [w375 w377]
          tunnel: [w374 w376] -> w369
          frame "Idle", Default {
            n150 = call <vilib>:"Unset Busy.vi"("error in (no error)"=w375) -> ("error out"=w374:errorcluster)  [unwired: 10 in]
          }
          frame "Busy" {
            n151 = call <vilib>:"Set Busy.vi"("error in (no error)"=w377) -> ("error out"=w376:errorcluster)  [unwired: 9 in, 1 out]
          }
        }
        n152 = call <vilib>:"Add State(s) to Queue__JKI_lib_State_Machine.vi"("State(s) in (\"\")"=w373) -> ("States Out"=w372:string)  [unwired: 14 in]
      }
      frame "UI: Front Panel State" {
        # "Argument"
        # "Set Front Panel Open or Closed\n(Usage: \"UI: Front Panel State >> Open|Close\")"
        n153 = Unbundle By Name(w381) -> ("Core.Current VI Reference"=w380:refnum<vi>)
        n154 = case shown="\"Open\", Default" w379 {
          tunnel: w383 -> [w389 w402]
          tunnel: [w391 w403] -> w382
          tunnel: w380 -> [w390 w400]
          frame "Open", Default {
            n155 = property class="VI"(reference=w390, error in=w389) -> (reference out=w387:refnum<vi>, error out=w388:errorcluster, "Front Panel.Open"=w386:bool)
            n156 = case shown="False" w386 {
              tunnel: [w394 w397] -> w391
              tunnel: w388 -> [w393 w397]
              tunnel: w387 -> [w392 _]
              frame False {
                n157 = invoke class="VI" method="FP.Open"(reference=w392, error in=w393, "Activate"=TRUE, "State"=T3."Standard") -> (error out=w394:errorcluster)  [unwired: 1 in, 4 out]
              }
              frame True {
              }
            }
          }
          frame "Close" {
            n158 = property class="VI"(reference=w400, error in=w402) -> (reference out=w399:refnum<vi>, error out=w401:errorcluster, "Front Panel.Open"=w398:bool)
            n159 = case shown="True" w398 {
              tunnel: [w404 w407] -> w403
              tunnel: w401 -> [w404 w406]
              tunnel: w399 -> [_ w405]
              frame False {
              }
              frame True {
                n160 = invoke class="VI" method="FP.Close"(reference=w405, error in=w406) -> (error out=w407:errorcluster)  [unwired: 1 in, 2 out]
              }
            }
          }
        }
        n161 = call <vilib>:"Add State(s) to Queue__JKI_lib_State_Machine.vi"("State(s) in (\"\")"=w385) -> ("States Out"=w384:string)  [unwired: 14 in]
      }
      frame "---------- Macro ----------" {
        n162 = call <vilib>:"Add State(s) to Queue__JKI_lib_State_Machine.vi"("State(s) in (\"\")"=w412) -> ("States Out"=w411:string)  [unwired: 14 in]
      }
      frame "Macro: Initialize" {
        n163 = call <vilib>:"Add State(s) to Queue__JKI_lib_State_Machine.vi"("State(s) in Front (\"\")"="Data: Initialize\nInitialize Core Data\nLaunch Handshake", "State(s) in (\"\")"=w418) -> ("States Out"=w417:string)  [unwired: 13 in]
      }
      frame "Macro: Exit" {
        n164 = Unbundle By Name(w429) -> ("Core.Close Panel on Exit?"=w428:bool)
        n165 = Flush Event Queue(0:w419, 3:w421) -> (11:w420:errorcluster)  [unwired: 4 in, 2 out]
        n166 = Select(t="UI: Front Panel State >> Close", s=w428, f="") -> (s? t:f=w425:string)
        n167 = call <vilib>:"Add State(s) to Queue__JKI_lib_State_Machine.vi"("State(s) in (\"\")"=w425, "State(s) at Back (\"\")"="Stop >> Stop with Exit\nSend Child Exit\nData: Cleanup\nExit") -> ("States Out"=w423:string)  [unwired: 13 in]
        n168 = call <vilib>:"Add State(s) to Queue__JKI_lib_State_Machine.vi"("State(s) in Front (\"\")"=w423, "State(s) in (\"\")"=w431) -> ("States Out"=w430:string)  [unwired: 13 in]
      }
      frame "---------- System state ----------" {
        n169 = call <vilib>:"Add State(s) to Queue__JKI_lib_State_Machine.vi"("State(s) in (\"\")"=w436) -> ("States Out"=w435:string)  [unwired: 14 in]
      }
      frame "Camera Info Requested" {
        n170 = in-place {
          in-place-border: w441 -> [w448]
          in-place-border: [w447] -> w440
          n171 = in-place-cluster #9(w439) -> ("Enqueuer.Nested Actor's Enqueuer"=w446:refnum<class "Message Enqueuer.lvclass">[], "CameraControllerParameters.CameraControllerParameters.CameraID"=w445:i32[], "Active Camera ID"=w444:i32[])
          n172 = for {
            shift-right: [w452] -> w447
            shift-left: w448 -> [w453]
            tunnel: w444 -> [w457] mode=indexing
            tunnel: w445 -> [w456]
            tunnel: w446 -> [w454]
            n173 = Search 1D Array(1D array=w456, element=w457) -> (index of element=w455:i32)  [unwired: 1 in]
            n174 = Index Array(array=w454, index=w455) -> (element=w450:refnum<class "Message Enqueuer.lvclass">)
            n175 = call "Send State Message IA.vi"("Message Priority (Normal)"=Message_Priority."High", "error in (no error)"=w453, "State Message"="Camera Info", "Message Enqueuer"=w450) -> ("error out"=w452:errorcluster)  [unwired: 6 in, 1 out]
          }
          n176 = in-place-cluster #9("Enqueuer.Nested Actor's Enqueuer"=w446, "CameraControllerParameters.CameraControllerParameters.CameraID"=w445, "Active Camera ID"=w444) -> (w438:T7)
        }
        n177 = call <vilib>:"Add State(s) to Queue__JKI_lib_State_Machine.vi"("State(s) in (\"\")"=w443) -> ("States Out"=w442:string)  [unwired: 14 in]
      }
      frame "Part Selected" {
        # "Number of Active Camera\n in each reciever"
        n178 = Unbundle By Name(w464) -> ("CameraControllerParameters.CameraControllerParameters.PartsList"=w479:T16, "CameraControllerParameters.PartName"=w481:string[])
        n179 = Unbundle By Name(w464) -> ("Enqueuer.Nested Actor's Enqueuer"=w462:refnum<class "Message Enqueuer.lvclass">[], "CameraControllerParameters.CameraControllerParameters.CameraID"=w463:i32[])
        n180 = Search 1D Array(1D array=w481, element=w459) -> (index of element=w480:i32)  [unwired: 1 in]
        n181 = Index Array(array=w479, index=w480) -> (element=w476:T17)
        n182 = Unbundle By Name(w476) -> ("PartName"=w475:string, "CameraIDs"=w461:i32[], "ReceiverSequence"=w460:T14)
        n183 = for {
          tunnel: [w496] -> w474 mode=indexing
          tunnel: [w501] -> w472 mode=indexing
          tunnel: w460 -> [w499] mode=indexing
          tunnel: [w493] -> w471 mode=indexing
          tunnel: [w498] -> w470 mode=indexing
          tunnel: [w496] -> w473
          tunnel: [w497] -> w469
          tunnel: [w492] -> w458
          w498 = u64 0  # Initial Value
          w500 = 0  # Initial Value
          w502 = T8 refnum  # Image Constants
          # "Based on the number of reciever in the CCA, Image array, Number of active camera, Image Revieved count and image count are Initialized"
          n184 = Unbundle By Name(w499) -> ("NoOfActiveCameras"=w493:i32)
          n185 = Initialize Array(cluster{"State":string, "Status":string} {"State"="", "Status"=""} ("Status Ack"), w493) -> (w492:cluster{"State":string, "Status":string}[])
          n186 = Initialize Array(T2 {"Camera Id"=0, "Camera Name"="", "Exposure Time"=0, "AOI"=[]} ("Camera Information"), w493) -> (w497:T13)
          n187 = Initialize Array(w502, w493) -> (w496:T8[])
          n188 = Initialize Array(w500, w493) -> (w501:i32[])
        }
        n189 = for {
          shift-right: [w490] -> w465
          shift-left: w466 -> [w491]
          tunnel: w463 -> [w489]
          tunnel: w462 -> [w486]
          tunnel: w461 -> [w488] mode=indexing
          tunnel: w459 -> [w484]
          n190 = Search 1D Array(1D array=w489, element=w488) -> (index of element=w487:i32)  [unwired: 1 in]
          n191 = Index Array(array=w486, index=w487) -> (element=w485:refnum<class "Message Enqueuer.lvclass">)
          n192 = call "Send Part Name IA.vi"("error in (no error)"=w491, "Part Name"=w484, "Message Enqueuer"=w485) -> ("error out"=w490:errorcluster)  [unwired: 7 in, 1 out]
        }
        n193 = call <vilib>:"Add State(s) to Queue__JKI_lib_State_Machine.vi"("State(s) in (\"\")"=w483) -> ("States Out"=w482:string)  [unwired: 14 in]
        n194 = Bundle By Name(cluster=w464, "CurrentPartDetails"=w476, "Part name"=w475, "Active Camera ID"=w461, "CurrentReceiverSequence"=w460, "Image array"=w474, "Output Data.Image Array"=w473, "Image count array"=w472, "Number of active cameras"=w471, "Images Recieved count"=w470, "Image Array Counter"=0, "All Camera Diagnostics"=FALSE, "Output Data.Camera Information"=w469, "Status Ack"=w458) -> (w477:T7)
      }
      frame "Override Camera Settings" {
        n195 = in-place {
          in-place-border: w507 -> [w512]
          in-place-border: [w511] -> w506
          n196 = in-place-cluster #10(w504) -> ("Enqueuer.Nested Actor's Enqueuer"=w515:refnum<class "Message Enqueuer.lvclass">[], "CameraControllerParameters.CameraControllerParameters.CameraID"=w514:i32[], "Active Camera ID"=w513:i32[], "Camera Setup"=w510:cluster{"Camera ID":i32, "Exposure time":i32}[])
          n197 = for {
            shift-right: [w521] -> w511
            shift-left: w512 -> [w517]
            tunnel: w513 -> [w522] mode=indexing
            tunnel: w514 -> [w526]
            tunnel: w515 -> [w525]
            tunnel: w510 -> [w524]
            n198 = Search 1D Array(1D array=w526, element=w522) -> (index of element=w523:i32)  [unwired: 1 in]
            n199 = for {
              tunnel: [w528] -> w518 if=w530
              tunnel: w524 -> [w529] mode=indexing
              tunnel: w522 -> [w531]
              stop <- w530 stop-if-true
              n200 = Unbundle By Name(w529) -> ("Exposure time"=w528:i32, "Camera ID"=w527:i32)
              n201 = Equal?(x=w527, y=w531) -> (x = y?=w530:bool)
            }
            n202 = Index Array(array=w525, index=w523) -> (element=w520:refnum<class "Message Enqueuer.lvclass">)
            n203 = Bundle By Name(cluster=cluster{"Exposure Time":i32} {"Exposure Time"=0} ("Camera Setup"), "Exposure Time"=w518) -> (w516:cluster{"Exposure Time":i32})
            n204 = call "Send Camera Setup IA.vi"("error in (no error)"=w517, "Camera Setup"=w516, "Message Enqueuer"=w520) -> ("error out"=w521:errorcluster)  [unwired: 7 in, 1 out]
          }
          n205 = in-place-cluster #10("Enqueuer.Nested Actor's Enqueuer"=w515, "CameraControllerParameters.CameraControllerParameters.CameraID"=w514, "Active Camera ID"=w513, "Camera Setup"=w510) -> (w503:T7)
        }
        n206 = call <vilib>:"Add State(s) to Queue__JKI_lib_State_Machine.vi"("State(s) in (\"\")"=w509) -> ("States Out"=w508:string)  [unwired: 14 in]
      }
      frame "Run" {
        n207 = in-place {
          in-place-border: w537 -> [w546]
          in-place-border: [w545] -> w536
          n208 = in-place-cluster #11(w535) -> ("Run Info.State"=w540:string, "Enqueuer.Nested Actor's Enqueuer"=w544:refnum<class "Message Enqueuer.lvclass">[], "CameraControllerParameters.CameraControllerParameters.CameraID"=w543:i32[], "Active Camera ID"=w542:i32[], "Run Info.Image File path"=w541:cluster{"Path":path, "Camera ID":i32}[])  [unwired: 1 out]
          n209 = case shown="\"OneshotE\", \"OneshotP\"" w540 {
            tunnel: ["" "Merge Image" "DustCalculation" "Merge Image"] -> w539
            frame Default {
            }
            frame "ContinuousE", "ContinuousP" {
            }
            frame "CameraOpticsDiagnostics" {
            }
            frame "OneshotE", "OneshotP" {
            }
          }
          n210 = for {
            shift-right: [w559] -> w545
            shift-left: w546 -> [w551]
            tunnel: w542 -> [w552] mode=indexing
            tunnel: w543 -> [w558]
            tunnel: w544 -> [w557]
            tunnel: w541 -> [w554]
            n211 = Search 1D Array(1D array=w558, element=w552) -> (index of element=w553:i32)  [unwired: 1 in]
            n212 = for {
              tunnel: [w563] -> w555 if=w560
              tunnel: w554 -> [w564] mode=indexing
              tunnel: w552 -> [w561]
              stop <- w560 stop-if-true
              n213 = Unbundle By Name(w564) -> ("Path"=w563:path, "Camera ID"=w562:i32)
              n214 = Equal?(x=w562, y=w561) -> (x = y?=w560:bool)
            }
            n215 = Index Array(array=w557, index=w553) -> (element=w556:refnum<class "Message Enqueuer.lvclass">)
            n216 = call "Send Run IA.vi"("error in (no error)"=w551, "Image File Path (If Offline)"=w555, "Message Enqueuer"=w556) -> ("error out"=w559:errorcluster)  [unwired: 7 in, 1 out]
          }
          n217 = in-place-cluster #11("Current Steps"=w539, "Run Info.State"=w540, "Enqueuer.Nested Actor's Enqueuer"=w544, "CameraControllerParameters.CameraControllerParameters.CameraID"=w543, "Active Camera ID"=w542, "Run Info.Image File path"=w541) -> (w534:T7)
        }
        n218 = call <vilib>:"Add State(s) to Queue__JKI_lib_State_Machine.vi"("State(s) in (\"\")"="") -> ("States Out"=w538:string)  [unwired: 14 in]
      }
      frame "Pause" {
        n219 = in-place {
          in-place-border: w569 -> [w576]
          in-place-border: [w575] -> w568
          n220 = in-place-cluster #12(w566) -> ("Enqueuer.Nested Actor's Enqueuer"=w574:refnum<class "Message Enqueuer.lvclass">[], "CameraControllerParameters.CameraControllerParameters.CameraID"=w573:i32[], "Active Camera ID"=w572:i32[])
          n221 = for {
            shift-right: [w580] -> w575
            shift-left: w576 -> [w581]
            tunnel: w572 -> [w585] mode=indexing
            tunnel: w573 -> [w584]
            tunnel: w574 -> [w582]
            n222 = Search 1D Array(1D array=w584, element=w585) -> (index of element=w583:i32)  [unwired: 1 in]
            n223 = Index Array(array=w582, index=w583) -> (element=w578:refnum<class "Message Enqueuer.lvclass">)
            n224 = call "Send State Message IA.vi"("Message Priority (Normal)"=Message_Priority."High", "error in (no error)"=w581, "State Message"="Pause", "Message Enqueuer"=w578) -> ("error out"=w580:errorcluster)  [unwired: 6 in, 1 out]
          }
          n225 = in-place-cluster #12("Enqueuer.Nested Actor's Enqueuer"=w574, "CameraControllerParameters.CameraControllerParameters.CameraID"=w573, "Active Camera ID"=w572) -> (w565:T7)
        }
        n226 = call <vilib>:"Add State(s) to Queue__JKI_lib_State_Machine.vi"("State(s) in (\"\")"=w571) -> ("States Out"=w570:string)  [unwired: 14 in]
      }
      frame "Stop" {
        n227 = Flush Event Queue(0:w587, 3:w589) -> (11:w588:errorcluster)  [unwired: 4 in, 2 out]
        n228 = in-place {
          in-place-border: w588 -> [w613]
          in-place-border: [w612] -> w593
          in-place-border: w591 -> [w610]
          w597 = u64 0 ("Image Array Counter")
          n229 = in-place-cluster #13(w592) -> ("CameraControllerParameters.CameraControllerParameters.Diagnostics.DiagnosticReceiverSequence.ReceiverName"=w606:string, "CameraControllerParameters.CameraControllerParameters.Diagnostics.DiagnosticReceiverSequence.ReceiverID"=w605:i32, "CameraControllerParameters.CameraControllerParameters.NoOfCameras"=w604:i32, "Enqueuer.Nested Actor's Enqueuer"=w611:refnum<class "Message Enqueuer.lvclass">[], "CameraControllerParameters.CameraControllerParameters.CameraID"=w598:i32[], "Active Camera ID"=w601:i32[], "Active Light Camera Name"=w603:string)  [unwired: 4 out]
          n230 = Empty String/Path?(string/path=w603) -> (empty?=w602:bool)
          n231 = Select(t=w601, s=w602, f=w598) -> (s? t:f=w596:i32[])
          n232 = for {
            shift-right: [w617] -> w612
            shift-left: w613 -> [w618]
            tunnel: w596 -> [w622] mode=indexing
            tunnel: w598 -> [w621]
            tunnel: w611 -> [w619]
            tunnel: w610 -> [w614]
            n233 = Search 1D Array(1D array=w621, element=w622) -> (index of element=w620:i32)  [unwired: 1 in]
            n234 = Index Array(array=w619, index=w620) -> (element=w616:refnum<class "Message Enqueuer.lvclass">)
            n235 = call "Send State Message IA.vi"("Message Priority (Normal)"=Message_Priority."High", "error in (no error)"=w618, "State Message"=w614, "Message Enqueuer"=w616) -> ("error out"=w617:errorcluster)  [unwired: 6 in, 1 out]
          }
          n236 = Bundle("ReceiverName"=w606, "ReceiverID"=w605, "NoOfCameras"=w604) -> (w608:T15)  [unwired: 1 in]
          n237 = Build Array(w608) -> (w607:T18)
          n238 = in-place-cluster #13("CurrentReceiverSequence"=w607, "CameraControllerParameters.CameraControllerParameters.Diagnostics.DiagnosticReceiverSequence.ReceiverName"=w606, "CameraControllerParameters.CameraControllerParameters.Diagnostics.DiagnosticReceiverSequence.ReceiverID"=w605, "CameraControllerParameters.CameraControllerParameters.NoOfCameras"=w604, "Current Steps"="", "Enqueuer.Nested Actor's Enqueuer"=w611, "CameraControllerParameters.CameraControllerParameters.CameraID"=w598, "Active Camera ID"=w596, "Active Light Camera Name"="", "Run Info"=T5 {"State"="", "Image File path"=[]}, "Image Array Counter"=w597) -> (w586:T7)
          n239 = global write "Image Trigger Global Count.vi" "Image Trigger Count"(w597) -> ()
        }
        n240 = call <vilib>:"Add State(s) to Queue__JKI_lib_State_Machine.vi"("State(s) in (\"\")"=w595) -> ("States Out"=w594:string)  [unwired: 14 in]
      }
      frame "Send Child Exit" {
        n241 = in-place {
          in-place-border: w627 -> [w635]
          in-place-border: [w634] -> w626
          n242 = in-place-cluster #14(w625) -> ("Enqueuer.Nested Actor's Enqueuer"=w633:refnum<class "Message Enqueuer.lvclass">[], "CameraControllerParameters.CameraControllerParameters.CameraID"=w630:i32[])  [unwired: 3 out]
          n243 = for {
            shift-right: [w637] -> w634
            shift-left: w635 -> [w638]
            tunnel: w630 -> [w642] mode=indexing
            tunnel: w630 -> [w641]
            tunnel: w633 -> [w639]
            n244 = Search 1D Array(1D array=w641, element=w642) -> (index of element=w640:i32)  [unwired: 1 in]
            n245 = Index Array(array=w639, index=w640) -> (element=w636:refnum<class "Message Enqueuer.lvclass">)
            n246 = call <vilib>:"Send Normal Stop.vi"("error in (no error)"=w638, "Message Enqueuer"=w636) -> ("error out"=w637:errorcluster)  [unwired: 9 in]
          }
          n247 = in-place-cluster #14("Current Steps"="", "Enqueuer.Nested Actor's Enqueuer"=w633, "CameraControllerParameters.CameraControllerParameters.CameraID"=w630, "Active Camera ID"=w630, "Active Light Camera Name"="") -> (w624:T7)
        }
        n248 = call <vilib>:"Add State(s) to Queue__JKI_lib_State_Machine.vi"("State(s) in (\"\")"=w629) -> ("States Out"=w628:string)  [unwired: 14 in]
      }
      frame "-----------Child Launch--------" {
        n249 = call <vilib>:"Add State(s) to Queue__JKI_lib_State_Machine.vi"("State(s) in (\"\")"=w647) -> ("States Out"=w646:string)  [unwired: 14 in]
      }
      frame "Launch Handshake" {
        n250 = call <vilib>:"Read Self Enqueuer.vi"("Actor"=w650) -> ("Self Enqueuer"=w652:refnum<class "Message Enqueuer.lvclass">)  [unwired: 10 in]
        n251 = control-ref of="This VI"() -> (w651:refnum<vi>)
        n252 = Unbundle By Name(w648) -> ("Output Data"=w655:T9)
        n253 = Bundle By Name(cluster=w655, "Launch Handshake.Actor Enqueuer Refnum"=w652, "Launch Handshake.Actor core Refnum"=w651) -> (w654:T9)
        n254 = call "ZenCAM Output.vi"("error in (no error)"=w657, "Output Data"=w654, "State"="Launch Handshake", "Camera Controller in"=w650) -> ("error out"=w656:errorcluster, "Camera Controller out"=w649:refnum<class "Camera Controller.lvclass">)  [unwired: 6 in]
        n255 = call <vilib>:"Add State(s) to Queue__JKI_lib_State_Machine.vi"("State(s) in (\"\")"=w659) -> ("States Out"=w658:string)  [unwired: 14 in]
      }
      frame "Launch Child Actor" {
        w671 = refnum<class "Image Acquisition.lvclass"> refnum  # Image Acquisition.lvclass
        n256 = Unbundle By Name(w662) -> ("CameraControllerParameters.CameraControllerParameters.CameraID"=w669:i32[], "CameraControllerParameters.CameraControllerParameters.NoOfCameras"=w670:i32)
        n257 = for {
          N: w670 -> [w678]
          shift-right: [w684] -> w672
          shift-left: w673 -> [w685]
          tunnel: w671 -> [w683]
          tunnel: w660 -> [w682]
          tunnel: [w679] -> w668 mode=indexing
          tunnel: [w678] -> w667 mode=indexing
          tunnel: [w677] -> w666 mode=indexing
          tunnel: [w676] -> w665 mode=indexing
          w676 = u64 0  # Initial Value
          w681 = 0  # Initial Value
          w680 = T8 refnum  # Image Constants
          n258 = call <vilib>:"Launch Nested Actor.vi"("error in (no error)"=w685, "Nested Actor"=w683, "Caller Actor in"=w682) -> ("error out"=w684:errorcluster)  [unwired: 6 in, 2 out]
          n259 = Initialize Array(w680, w678) -> (w679:T8[])
          n260 = Initialize Array(w681, w678) -> (w677:i32[])
        }
        n261 = Bundle By Name(cluster=w662, "Active Camera ID"=w669, "Image array"=w668, "Number of active cameras"=w667, "Image count array"=w666, "Images Recieved count"=w665, "Image Array Counter"=u64 0, "All Camera Diagnostics"=FALSE ("OneShot?")) -> (w661:T7)
        n262 = call <vilib>:"Add State(s) to Queue__JKI_lib_State_Machine.vi"("State(s) in (\"\")"=w675) -> ("States Out"=w674:string)  [unwired: 14 in]
      }
      frame "Send Child ID" {
        n263 = Unbundle By Name(w688) -> ("CC Json File Path"=w687:path)
        n264 = Unbundle By Name(w691) -> ("Enqueuer.Nested Actor's Enqueuer"=w690:refnum<class "Message Enqueuer.lvclass">[], "CameraControllerParameters.CameraControllerParameters.CameraID"=w689:i32[])
        n265 = for {
          shift-right: [w695] -> w692
          shift-left: w693 -> [w696]
          tunnel: w690 -> [w701] mode=indexing
          tunnel: w689 -> [w699] mode=indexing
          tunnel: w687 -> [w698]
          n266 = Bundle By Name(cluster=T6 {"Image Acquisition ID"=0, "IA JSON File Path"=path ""} ("Image Acquisition Setup"), "Image Acquisition ID"=w699, "IA JSON File Path"=w698) -> (w697:T6)
          n267 = call "Send Image Acqusition Setup IA.vi"("error in (no error)"=w696, "Image Acquisition Setup"=w697, "Message Enqueuer"=w701) -> ("error out"=w695:errorcluster)  [unwired: 7 in, 1 out]
        }
        n268 = call <vilib>:"Add State(s) to Queue__JKI_lib_State_Machine.vi"("State(s) in (\"\")"="Launch Successful" ("State(s) in Front (\"\")")) -> ("States Out"=w694:string)  [unwired: 14 in]
      }
      frame "Launch Successful" {
        n269 = Unbundle By Name(w705) -> ("Output Data"=w704:T9)
        n270 = Bundle By Name(cluster=w704, "Launch Clear"=TRUE) -> (w702:T9)
        n271 = call "ZenCAM Output.vi"("error in (no error)"=w710, "Output Data"=w702, "State"="Launch Successful", "Camera Controller in"=w708) -> ("error out"=w709:errorcluster, "Camera Controller out"=w707:refnum<class "Camera Controller.lvclass">)  [unwired: 6 in]
        n272 = call <vilib>:"Add State(s) to Queue__JKI_lib_State_Machine.vi"("State(s) in (\"\")"=w712) -> ("States Out"=w711:string)  [unwired: 14 in]
      }
      frame "---------- Diagnostics ----------" {
        n273 = call <vilib>:"Add State(s) to Queue__JKI_lib_State_Machine.vi"("State(s) in (\"\")"=w717) -> ("States Out"=w716:string)  [unwired: 14 in]
      }
      frame "Camera Optics Diagnostics" {
        n274 = case shown="\"OFF\"" w719 {
          tunnel: w722 -> [w727 w733 w736]
          tunnel: [w726 w733 w735] -> w721
          tunnel: ["" "" "Run" ("State(s) in (\"\")")] -> w718
          frame "OFF" {
            n275 = in-place {
              n276 = in-place-cluster #15(w727) -> ("CameraControllerParameters.CameraControllerParameters.Diagnostics.LightCameraSequence"=w731:T19, "CameraControllerParameters.CameraControllerParameters.CameraID"=w730:i32[])  [unwired: 3 out]
              n277 = in-place-cluster #15("Run Info.State"="", "CameraControllerParameters.CameraControllerParameters.Diagnostics.LightCameraSequence"=w731, "Active Light Camera Name"="", "CameraControllerParameters.CameraControllerParameters.CameraID"=w730, "Active Camera ID"=w730) -> (w726:T7)
            }
          }
          frame Default {
          }
          frame "ON" {
            n278 = in-place {
              n279 = in-place-cluster #16(w736) -> ("CameraControllerParameters.CameraControllerParameters.Diagnostics.LightCameraSequence"=w740:T19, "Active Light Camera Name"=w739:string)  [unwired: 2 out]
              n280 = for {
                tunnel: w740 -> [w743] mode=indexing
                tunnel: [w745] -> w738 mode=indexing if=w744
                tunnel: w739 -> [w742]
                i -> [w745]
                stop <- w744 stop-if-true
                n281 = Unbundle By Name(w743) -> ("Name"=w741:string)
                n282 = Equal?(x=w741, y=w742) -> (x = y?=w744:bool)
              }
              n283 = in-place-cluster #16("Run Info.State"="CameraOpticsDiagnostics", "CameraControllerParameters.CameraControllerParameters.Diagnostics.LightCameraSequence"=w740, "Active Light Camera Name"=w739, "Active Camera ID"=w738) -> (w735:T7)
            }
          }
        }
        n284 = call <vilib>:"Add State(s) to Queue__JKI_lib_State_Machine.vi"("State(s) in (\"\")"=w718) -> ("States Out"=w724:string)  [unwired: 14 in]
      }
      frame "DustCalculation" {
        n285 = Unbundle By Name(w753) -> ("Output Data"=w752:T9, "Active Light Camera Name"=w755:string, "CameraControllerParameters"=w760:T10, "Captured Image Info.Image out"=w759:T8)
        n286 = call "DiagnosticCheckMain.vi"("CameraControllerParameters.Diagnostics"=w760, "Diagnostic Check Image"=w759, "error in (no error)"=w754) -> ("Diagnostics Passed"=w758:bool, "Diagnostic Check Image out"=w757:T8, "Dust Percentage"=w756:dbl, "error out"=w751:errorcluster)  [unwired: 8 in, 1 out]
        n287 = Bundle By Name(cluster=w752, "CamOpticsDiagnosticsResult.Light Camera  Name"=w755, "CamOpticsDiagnosticsResult.Result"=w758, "CamOpticsDiagnosticsResult.Diagnosed Image"=w757, "CamOpticsDiagnosticsResult.Dust Percentage"=w756) -> (w746:T9)
        n288 = call "ZenCAM Output.vi"("error in (no error)"=w751, "Output Data"=w746, "State"="COD Result", "Camera Controller in"=w749) -> ("error out"=w750:errorcluster, "Camera Controller out"=w748:refnum<class "Camera Controller.lvclass">)  [unwired: 6 in]
        n289 = call <vilib>:"Add State(s) to Queue__JKI_lib_State_Machine.vi"("State(s) in (\"\")"=w762) -> ("States Out"=w761:string)  [unwired: 14 in]
      }
      frame "---------- Image Handing---------" {
        n290 = call <vilib>:"Add State(s) to Queue__JKI_lib_State_Machine.vi"("State(s) in (\"\")"=w767) -> ("States Out"=w766:string)  [unwired: 14 in]
      }
      frame "Merge Image" {
        n291 = call "Merge Image.vi"("error in (no error)"=w777, "Camera Control Cluster"=w773, "Camera Controller in"=w774) -> ("error out"=w776:errorcluster, "Camera Control Cluster Out"=w772:T7, "Camera Controller out"=w775:refnum<class "Camera Controller.lvclass">)  [unwired: 6 in]
        n292 = Unbundle By Name(w772) -> ("Image Array Counter"=w768:u64)
        "Image Array Counter" <- w768
        n293 = Unbundle By Name(w773) -> ("Image Array Counter"=w769:u64, "Run Info.State"=w771:string)
        n294 = case shown="\"OneshotE\", \"OneshotP\"" w771 {
          tunnel: ["" w780] -> w770
          tunnel: w768 -> [_ w784]
          tunnel: w769 -> [_ w783]
          frame Default {
          }
          frame "OneshotE", "OneshotP" {
            n295 = Equal?(x=w784, y=w783) -> (x = y?=w785:bool)
            n296 = Select(t="", s=w785, f="Stop >> Stop") -> (s? t:f=w780:string)
          }
        }
        n297 = call <vilib>:"Add State(s) to Queue__JKI_lib_State_Machine.vi"("State(s) in (\"\")"=w770) -> ("States Out"=w778:string)  [unwired: 14 in]
      }
      frame "---------- Camera Information---------" {
        n298 = call <vilib>:"Add State(s) to Queue__JKI_lib_State_Machine.vi"("State(s) in (\"\")"=w790) -> ("States Out"=w789:string)  [unwired: 14 in]
      }
      frame "Send Merged Camera Information" {
        n299 = Unbundle By Name(w799) -> ("Active Camera ID"=w795:i32[], "Output Data"=w793:T9)
        n300 = Array Size(array=w795) -> (size(s)=w794:i32)
        n301 = Initialize Array(T2 {"Camera Id"=0, "Camera Name"="", "Exposure Time"=0, "AOI"=[]} ("Camera Information"), w794) -> (w796:T13)
        n302 = Bundle By Name(cluster=w793, "Number of Active Camera"=w794) -> (w792:T9)
        n303 = Bundle By Name(cluster=w799, "Output Data.Camera Information"=w796, "Camera Info Recieved"=0) -> (w798:T7)
        n304 = call "ZenCAM Output.vi"("error in (no error)"=w804, "Output Data"=w792, "State"="Send Camera Info", "Camera Controller in"=w802) -> ("error out"=w803:errorcluster, "Camera Controller out"=w801:refnum<class "Camera Controller.lvclass">)  [unwired: 6 in]
        n305 = call <vilib>:"Add State(s) to Queue__JKI_lib_State_Machine.vi"("State(s) in (\"\")"=w806) -> ("States Out"=w805:string)  [unwired: 14 in]
      }
      frame "Send State Ack" {
        n306 = Unbundle By Name(w821) -> ("Active Camera ID"=w815:i32[], "Output Data"=w813:T9, "Status Ack"=w812:cluster{"State":string, "Status":string}[])
        n307 = Array Size(array=w815) -> (size(s)=w814:i32)
        n308 = for {
          tunnel: w812 -> [w833] mode=indexing
          tunnel: [w830] -> w810
          tunnel: [w829] -> w811
          stop <- w830 continue-if-true
          n309 = Unbundle By Name(w833) -> ("State"=w829:string, "Status"=w832:string)
          n310 = Equal?(x=w832, y="Done") -> (x = y?=w830:bool)
        }
        n311 = Initialize Array(cluster{"State":string, "Status":string} {"State"="", "Status"=""} ("Status Ack"), w814) -> (w819:cluster{"State":string, "Status":string}[])
        n312 = Bundle By Name(cluster=w821, "Status Ack"=w819, "Setup Response Received Count"=0) -> (w820:T7)
        n313 = Select(t="Done", s=w810, f="Fail") -> (s? t:f=w807:string)
        n314 = Bundle By Name(cluster=w813, "State Ack.State Message"=w811, "State Ack.Status"=w807) -> (w818:T9)
        n315 = call "ZenCAM Output.vi"("error in (no error)"=w826, "Output Data"=w818, "State"="Send State Ack", "Camera Controller in"=w824) -> ("error out"=w825:errorcluster, "Camera Controller out"=w823:refnum<class "Camera Controller.lvclass">)  [unwired: 6 in]
        n316 = call <vilib>:"Add State(s) to Queue__JKI_lib_State_Machine.vi"("State(s) in (\"\")"=w828) -> ("States Out"=w827:string)  [unwired: 14 in]
      }
    }
  }
  n317 = call-parent "Actor Core.vi"("error in"="error in", "Actor in"="Camera Controller in") -> ("error out"=→"error out":errorcluster, "Actor out"=→"Actor out":refnum<class "Actor.lvclass">)  [unwired: 8 in]
